vi "LK340Status Settled.vi"(0 "VISA resource name":refnum<visa-resource-name>, 11 "error in (no error)":errorcluster) -> (4 "VISA resource name out":refnum<visa-resource-name>, 8 "Settled":bool, 15 "error out":errorcluster)   [LabVIEW 2015]
doc: "This VI may be used to verify the processing of a command has completed."
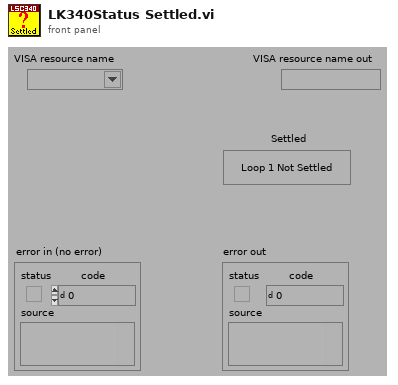
[diagram p1: front panel]
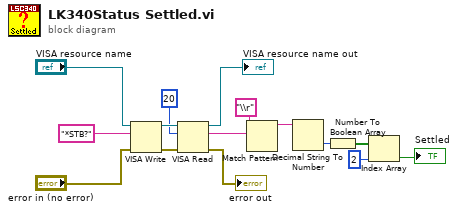
[diagram p0: block diagram]
diagram:
  n1 = VISA Write(VISA resource name="VISA resource name", write buffer="*STB?", error in (no error)="error in (no error)") -> (VISA resource name out=w15:refnum<visa-resource-name>, error out=w14:errorcluster)  [unwired: 1 out]
  n2 = VISA Read(VISA resource name=w15, byte count=20, error in (no error)=w14) -> (VISA resource name out=→"VISA resource name out":refnum<visa-resource-name>, read buffer=w12:string, error out=→"error out":errorcluster)  [unwired: 1 out]
  n3 = Match Pattern(string=w12, regular expression="\\r") -> (before substring=w5:string)  [unwired: 4 out]
  n4 = Decimal String To Number(string=w5) -> (number=w4:i32)  [unwired: 3 out]
  n5 = Number To Boolean Array(number=w4) -> (Boolean array=w3:bool[])
  n6 = Index Array(array=w3, index=2) -> (element=→"Settled":bool)
